vi "LIA_FPGA.vi"() -> ()   [LabVIEW 2012]
uses:
  <vilib>/rvi/DataTransferAndStorage/Container/Common/niFpgaContainerMetaDataKey.ctl
  <vilib>/rvi/DataTransferAndStorage/Container/Common/niFpgaContainerState.ctl
  <vilib>/rvi/DataTransferAndStorage/Container/Common/niFpgaDataTypeControl.ctl
  <vilib>/rvi/DataTransferAndStorage/Container/Common/niFpgaContainerImplementationControl.ctl
  <vilib>/rvi/DataTransferAndStorage/Container/Common/niFpgaContainerArbitrationOptionsControl.ctl
  <vilib>/rvi/DataTransferAndStorage/Container/Common/niFpgaTransferTypeControl.ctl
  <vilib>/rvi/DataTransferAndStorage/Container/Common/niFpgaContainerInitializationParameters.ctl
  <vilib>/rvi/Memory/Memory_Types/niFpgaMemoryInterfaceConfiguration.ctl
  <vilib>/rvi/FIFO/Fifo_Types/niFpgaFifoControlLogicControl.ctl
  <vilib>/rvi/FXPMathLib/FxpSinAndCos/subVIs/nifxpmath_SinAndCos_SimConfig.ctl
  <vilib>/rvi/DataTransferAndStorage/Container/Common/niFpgaContainerGetUniqueNameForEmu.vi
  <vilib>/rvi/DataTransferAndStorage/Container/Common/niFpgaContainerSetEmuInfo.vi
  <vilib>/rvi/eio/common/nirviEmuReportErrorAndStop.vi
  <vilib>/rvi/Emulation/niFpgaSctlEmulationGetInTimedLoop.vi
  <vilib>/rvi/FIFO/Fifo_Resource/nirvififoEmulationSetSize.vi
  <vilib>/rvi/Emulation/niFpgaSctlEmulationFifoFullMgr.vi
  <vilib>/rvi/errors/niFpgaSetErrorForExecOnDevCompSimple.vi
  <vilib>/rvi/eio/common/nirviEmuTemplateMethod_errors.vi
  <vilib>/rvi/FXPMathLib/FxpSinAndCos/simVIs/DllFxpSinAndCosTemp_sub.vi
  <vilib>/rvi/Emulation/niFpgaSctlEmulationResourceMgr.vi
  <vilib>/rvi/interface/RandomDataEmulation/nirviRandomDataFPGAFIFO.vi
  <vilib>/rvi/interface/RandomDataEmulation/niFpgaRandomDataHandleErrors.vi
  <vilib>/rvi/LocalResourceManager/LocalResourceManager.xnode
  <vilib>/rvi/DataTransferAndStorage/Container/XNode/niFpgaContainer.xnode
  <vilib>/rvi/FIFO/Fifo_Resource/nirvififoEmulationRead.vi
  <vilib>/eio/EIONode/EIONode.xnode
  <vilib>/rvi/FXPMathLib/FxpSinAndCos/XNode/nifxpmath_SinAndCos.xnode
  <vilib>/rvi/FIFO/Fifo_Resource/nirvififoEmulationWrite.vi
  <vilib>/rvi/interface/RandomDataEmulation/nirviRandomDataFpgaReadWriteTemplate.vi
  <vilib>/Platform/TimedLoop/XDataNode/wakeup.ctl
  <vilib>/Platform/TimedLoop/XDataNode/XDNodeRunTimeDep.lvlib
  <vilib>/Platform/TimedLoop/XDataNode/nitl_modes.ctl
  <vilib>/Platform/TimedLoop/XDataNode/timing_clust.ctl
  <vilib>/Platform/TimedLoop/XDataNode/XDataNode.xnode
panel:
  in  "dec":i32
  out "channelQ":i64
  out "channelI":i64
  in  "reset":bool
  out "f_2":fxp<+/-,32,0> format="%.32g"
  out "f":fxp<+/-,32,0> format="%.32g"
  in  "test":bool
  out "error":bool
  in  "dec2":i16
  in  "K":fxp<+/-,16,1>
  in  "nominal freq":fxp<+/-,16,1>
  in  "dec1":i16
  in  "stages":i8=1
  in  "stop":bool
  in  "decimation":i16=1024
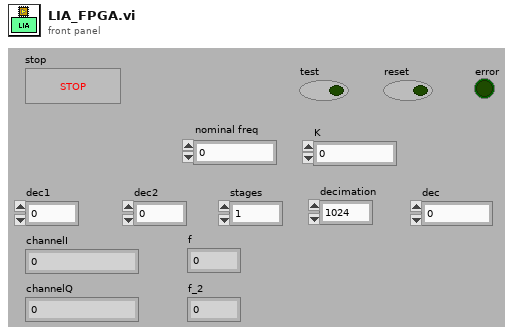
[diagram p1: front panel]
types:
  T1 = typedef "XDNodeRunTimeDep.lvlib/timing_clust.ctl" = cluster{"Expected End [f-1]":u64, "Actual End [f-1]":u64, "Finished Late? [f-1]":bool, "Expected End [i-1]":u64, "Actual End [i-1]":u64, "Finished Late? [i-1]":bool, "Expected Start [i]":u64, "Actual Start [i]":u64, "Expected Start [f]":u64, "Actual Start [f]":u64, "Source Name":string, "Structure Name":string, "Period":i64, "Deadline":i64, "Offset":i64, "Start":i64, "Priority":i32, "Timeout":i32, "Mode":T2, "Wakeup Reason":T3, "Error":errorcluster, "Source Type":string, "Secondary Source Type":string, "Global End Time":u64, "Global Start Time":u64, "Frame Duration":u64, "Iteration Duration":u64, "Assigned CPU":i32, "I/O Scan Engine Mode":u32}
  T2 = typedef "XDNodeRunTimeDep.lvlib/nitl_modes.ctl" = enum32{"No Change", "Process missed periods, maintain original phase", "Discard missed periods, maintain original phase", "Process missed periods, ignore original phase", "Discard missed periods, ignore original phase"}
  T3 = typedef "XDNodeRunTimeDep.lvlib/wakeup.ctl" = enum32{"Normal", "Aborted", "Asynchronous wakeup", "Timing source error", "Timed loop error", "Timeout"}
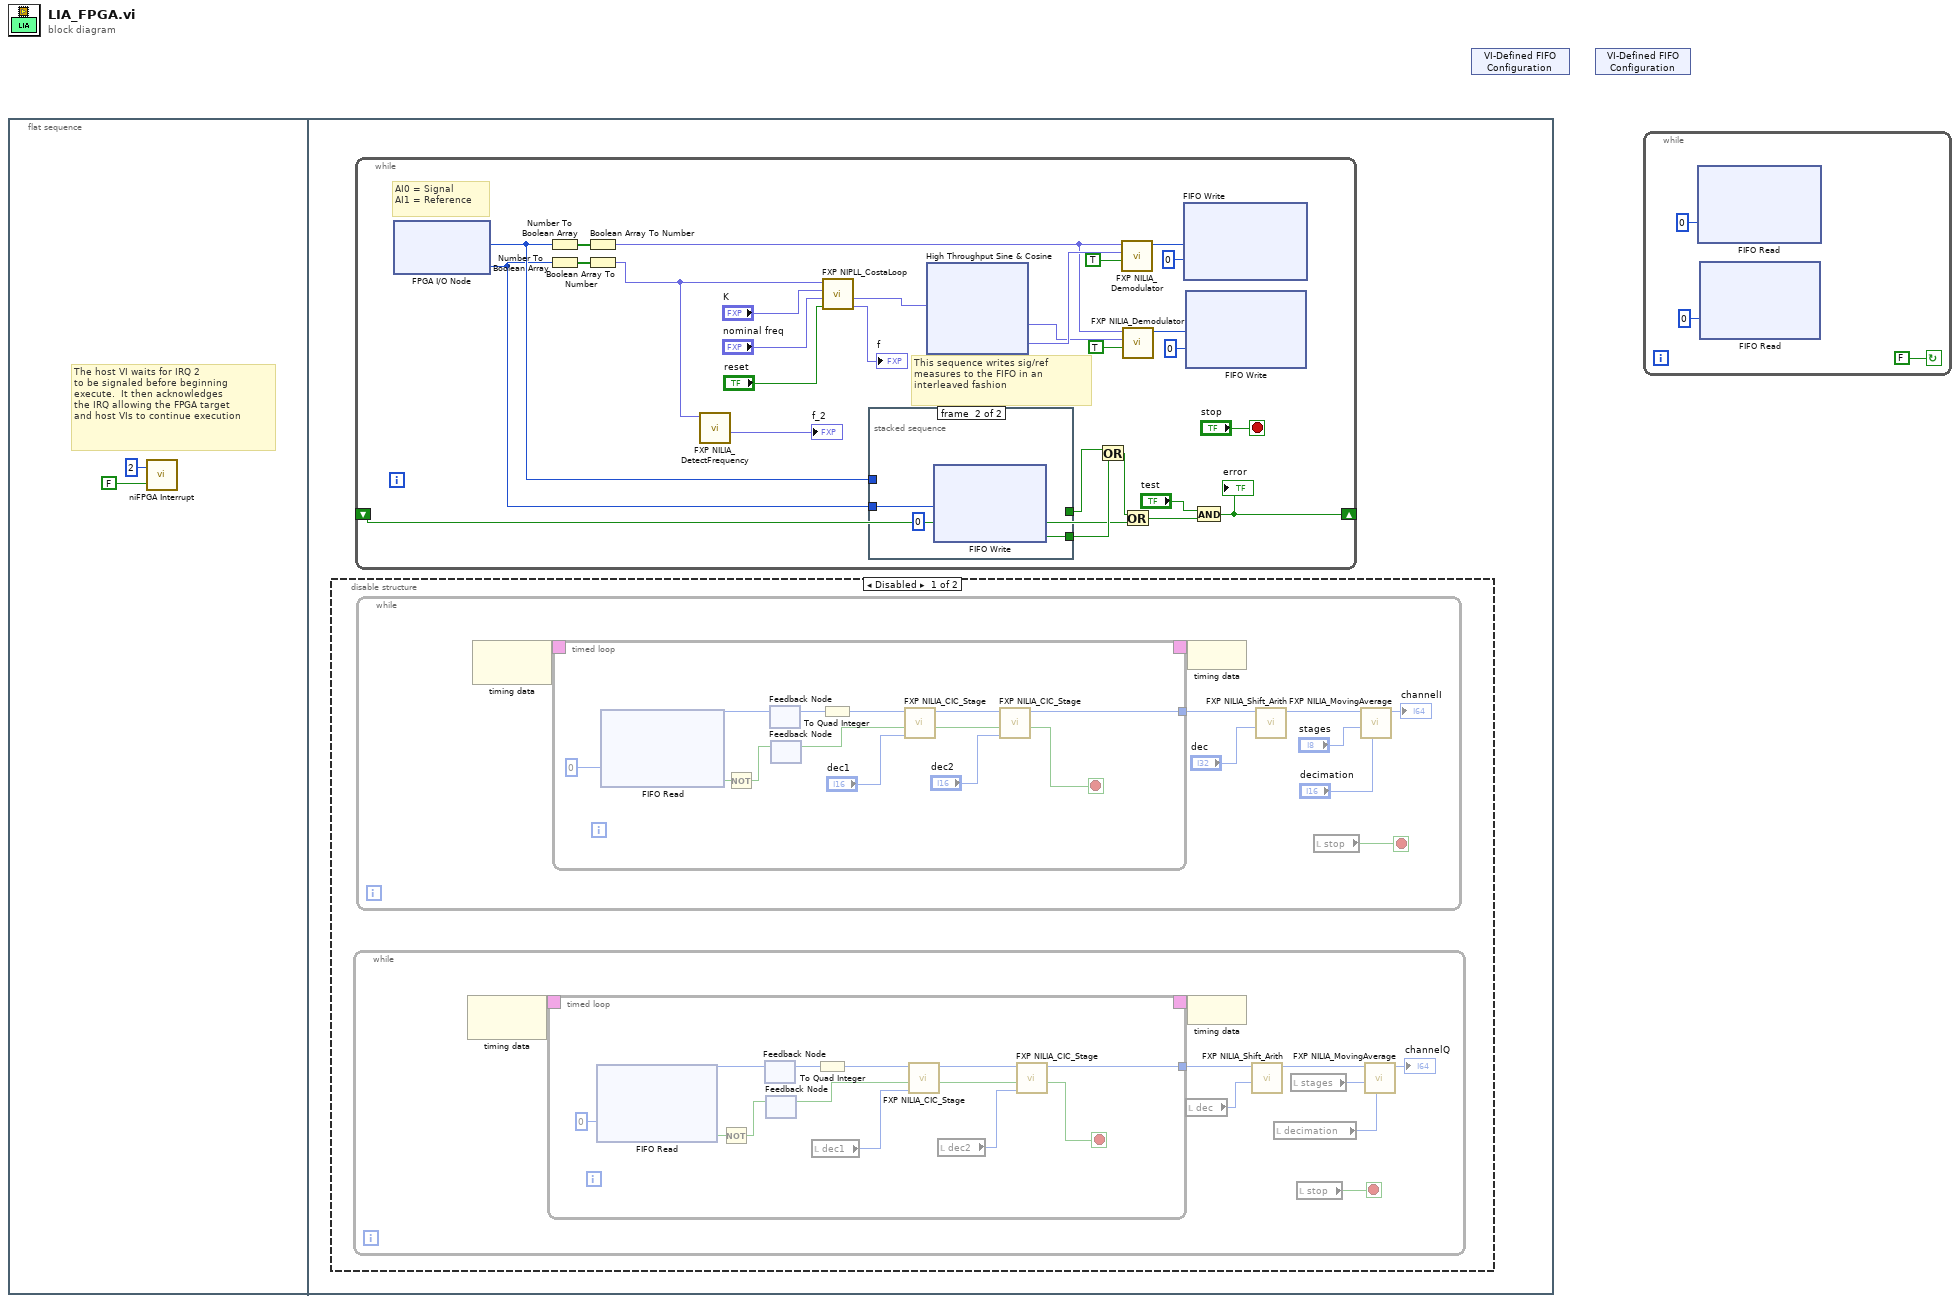
[diagram p0: block diagram]
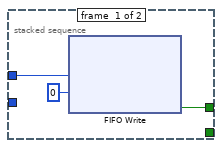
[diagram p3: hidden frame]
diagram:
  n1 = flat-sequence {
    frame #0 {
      # "The host VI waits for IRQ 2\nto be signaled before beginning\nexecute.  It then acknowledges\nthe IRQ allowing the FPGA target\nand host VIs to continue execution"
      n2 = call <vilib>:"niFPGA Interrupt.vi"("Wait Until Cleared (F)"=FALSE ("Wait Until Cleared"), "IRQ Number (0)"=u8 2 ("IRQ Number")) -> ()  [unwired: 1 in]
    }
    frame #1 {
      n3 = disable-structure shown="Disabled" {
        frame Disabled {
          n4 = while {
            stop <- w9 stop-if-true
            n5 = node-c288() -> (w11:T1)  [unwired: 1 in]
            n6 = timed-loop {
              timing: w11 -> [_]
              timing-out: [_] -> w10
              tunnel: [w13] -> w8
              stop <- w12 stop-if-true
              n7 = xnode ("FIFO Read")("Timeout"=0) -> ("Element"=w22:i32, "Timed Out?"=w21:bool)  [unwired: 1 in, 1 out]
              n8 = Not(x=w21) -> (.not. x?=w20:bool)
              n9 = feedback-in #1(w22) -> ()
              n10 = feedback #1() -> (w24:i32)  [unwired: 1 in]
              n11 = feedback-in #2(w20) -> ()
              n12 = feedback #2() -> (w18:bool)  [unwired: 1 in]
              n13 = local read "dec1"() -> (w17:i16)
              n14 = To Quad Integer(1:w24) -> (0:w19:i64)
              n15 = call "FXP NILIA_CIC_Stage.vi"("decimate factor"=w17, "New Data"=w18, "input"=w19) -> ("Data Ready"=w15:bool, "output"=w16:i64)  [unwired: 7 in]
              n16 = local read "dec2"() -> (w14:i16)
              n17 = call "FXP NILIA_CIC_Stage.vi"("decimate factor"=w14, "New Data"=w15, "input"=w16) -> ("Data Ready"=w12:bool, "output"=w13:i64)  [unwired: 7 in]
            }
            n18 = local read "dec"() -> (w7:i32)
            n19 = node-c288(w10) -> ()
            n20 = call "FXP NILIA_Shift_Arith.vi"("dec"=w7, "x"=w8) -> ("y"=w6:i64)  [unwired: 9 in]
            n21 = local read "decimation"() -> (w4:i16)
            n22 = local read "stages"() -> (w5:i8)
            n23 = local read "stop"() -> (w9:bool)
            n24 = call "FXP NILIA_MovingAverage.vi"("decimate"=w4, "stages"=w5, "input"=w6) -> ("output"=→"channelQ":i64)  [unwired: 8 in]
          }
          n25 = while {
            stop <- w35 stop-if-true
            n26 = node-c288() -> (w37:T1)  [unwired: 1 in]
            n27 = timed-loop {
              timing: w37 -> [_]
              timing-out: [_] -> w36
              tunnel: [w39] -> w34
              stop <- w38 stop-if-true
              n28 = xnode ("FIFO Read")("Timeout"=0) -> ("Element"=w48:i32, "Timed Out?"=w47:bool)  [unwired: 1 in, 1 out]
              n29 = Not(x=w47) -> (.not. x?=w46:bool)
              n30 = feedback-in #3(w48) -> ()
              n31 = feedback #3() -> (w50:i32)  [unwired: 1 in]
              n32 = feedback-in #4(w46) -> ()
              n33 = feedback #4() -> (w44:bool)  [unwired: 1 in]
              n34 = To Quad Integer(1:w50) -> (0:w45:i64)
              n35 = call "FXP NILIA_CIC_Stage.vi"("decimate factor"="dec1", "New Data"=w44, "input"=w45) -> ("Data Ready"=w41:bool, "output"=w42:i64)  [unwired: 7 in]
              n36 = call "FXP NILIA_CIC_Stage.vi"("decimate factor"="dec2", "New Data"=w41, "input"=w42) -> ("Data Ready"=w38:bool, "output"=w39:i64)  [unwired: 7 in]
            }
            n37 = node-c288(w36) -> ()
            n38 = call "FXP NILIA_Shift_Arith.vi"("dec"="dec", "x"=w34) -> ("y"=w32:i64)  [unwired: 9 in]
            n39 = local read "stop"() -> (w35:bool)
            n40 = call "FXP NILIA_MovingAverage.vi"("decimate"="decimation", "stages"="stages", "input"=w32) -> ("output"=→"channelI":i64)  [unwired: 8 in]
          }
        }
        frame Enabled {
        }
      }
      n41 = while {
        shift-right: [w74] -> _
        shift-left: _ -> [w76]
        stop <- "stop" stop-if-true
        # "This sequence writes sig/ref\nmeasures to the FIFO in an\ninterleaved fashion"
        # "AI0 = Signal\nAI1 = Reference"
        n42 = xnode "FPGA I/O Node"() -> ("Mod1/AI0"=w65:i16, "Mod1/AI1"=w64:i16)  [unwired: 2 in, 2 out]
        n43 = Number To Boolean Array(number=w65) -> (Boolean array=w67:bool[])
        n44 = Number To Boolean Array(number=w64) -> (Boolean array=w66:bool[])
        n45 = Boolean Array To Number(Boolean array=w67) -> (number=w58:fxp<+/-,24,1>)
        n46 = Boolean Array To Number(Boolean array=w66) -> (number=w63:fxp<+/-,24,1>)
        n47 = call "FXP NILIA_DetectFrequency.vi"("x"=w63) -> ("f_2"=→"f_2":fxp<+/-,32,0>)  [unwired: 9 in, 1 out]
        n48 = call "FXP NIPLL_CostaLoop.vi"("reset?"="reset", "norminal freq [U16.0]"="nominal freq", "alpha [U16.0]"="K", "x[I24.1]"=w63) -> ("f"=→"f":fxp<+/-,32,0>, "z [I32.1]"=w71:fxp<+/-,32,1>)  [unwired: 4 in, 2 out]
        n49 = stacked-sequence {
          tunnel: w65 -> [w114 _]
          tunnel: w64 -> [_ w117]
          tunnel: [w113 _] -> w80
          tunnel: [_ w116] -> w79
          frame #0 {
            n50 = xnode ("FIFO Write")("Element"=w114, "Timeout"=0) -> ("Timed Out?"=w113:bool)  [unwired: 1 in, 1 out]
          }
          frame #1 {
            n51 = xnode ("FIFO Write")("Element"=w117, "Timeout"=0) -> ("Timed Out?"=w116:bool)  [unwired: 1 in, 1 out]
          }
        }
        n52 = xnode "High Throughput Sine & Cosine"("x (pi)"=w71) -> ("sin(x)"=w57:fxp<+/-,24,2>, "cos(x)"=w61:fxp<+/-,24,2>)
        n53 = Or(x=w80, y=w79) -> (x .or. y?=w78:bool)
        n54 = call "FXP NILIA_Demodulator.vi"("New Data"=TRUE, "ref"=w61, "signal"=w58) -> ("x*y"=w59:i32)  [unwired: 7 in, 1 out]
        n55 = call "FXP NILIA_Demodulator.vi"("New Data"=TRUE, "ref"=w57, "signal"=w58) -> ("x*y"=w55:i32)  [unwired: 7 in, 1 out]
        n56 = Or(x=w78, y=w76) -> (x .or. y?=w77:bool)
        n57 = xnode ("FIFO Write")("Element"=w59, "Timeout"=0) -> ()  [unwired: 1 in, 2 out]
        n58 = xnode ("FIFO Write")("Element"=w55, "Timeout"=0) -> ()  [unwired: 1 in, 2 out]
        n59 = And(x="test", y=w77) -> (x .and. y?=w74:bool)
        "error" <- w74
      }
    }
  }
  n60 = xnode "VI-Defined FIFO Configuration"() -> ()  [unwired: 1 out]
  n61 = xnode "VI-Defined FIFO Configuration"() -> ()  [unwired: 1 out]
  n62 = while {
    stop <- FALSE continue-if-true
    n63 = xnode ("FIFO Read")("Timeout"=0) -> ()  [unwired: 1 in, 3 out]
    n64 = xnode ("FIFO Read")("Timeout"=0) -> ()  [unwired: 1 in, 3 out]
  }
